vi "Save and Close System Definition.vi"(8 "error in (no error)":errorcluster, 11 "SysDef Ref":T1) -> (0 "error out":errorcluster, 3 "SysDef Ref out":T1)   [LabVIEW 2019, in "Simple SysDef API.lvlib"]
uses:
  <userlib>/SimpleSysDef/Simple SysDef API.lvlib
  <userlib>/SimpleSysDef/_SubVIs/System Definition Reference.ctl
  NationalInstruments.VeriStand.SystemDefinitionAPI
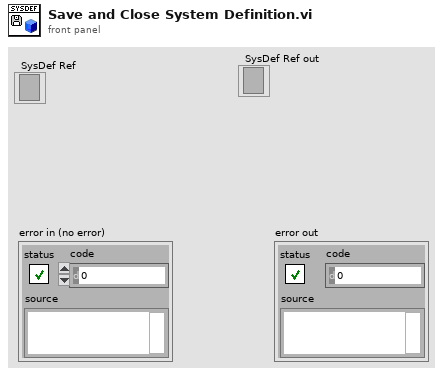
[diagram p1: front panel]
types:
  T1 = typedef "Simple SysDef API.lvlib/System Definition Reference.ctl" = refnum<k24>
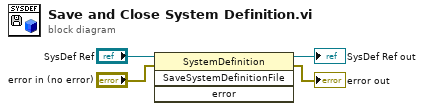
[diagram p0: block diagram]
diagram:
  n1 = invoke class="SystemDefinition" method="SaveSystemDefinitionFile"(reference="SysDef Ref", error in="error in (no error)") -> (reference out=→"SysDef Ref out":T1, error out=→"error out":errorcluster)  [unwired: 2 in, 2 out]
